vi "Unflatten.vi"(9 "VarTree_in":T1 {"Rawdata" format="0x%08x"}, 11 "In_Char":string) -> (0 "error out":errorcluster, 1 "VarTree_out":T1 {"Rawdata" format="0x%08x"}, 3 "Stat_Ok":bool)   [LabVIEW 2014]
uses:
  _init_vartree/typedefs/ExVarTreeArray.ctl
  _init_vartree/typedefs/ExVarTree.ctl
  _init_vartree/typedefs/val_type_t.ctl
panel:
  out "VarTree size(s)":i32
  out "Read size(s)":i32
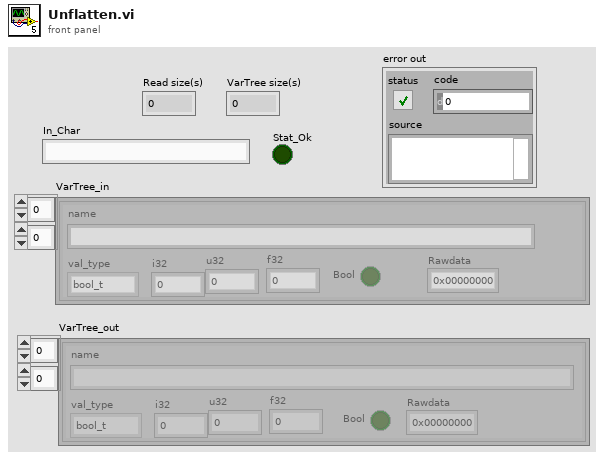
[diagram p1: front panel]
types:
  T1 = typedef "ExVarTreeArray.ctl" = T2[][]
  T2 = typedef "ExVarTree.ctl" = cluster{"name":string, "val_type":T3, "Rawdata":u32, "i32":i32, "u32":u32, "f32":sgl, "Bool":bool}
  T3 = typedef "val_type_t.ctl" = enum16{"bool_t", "i32_t", "u32_t", "f32_t"}
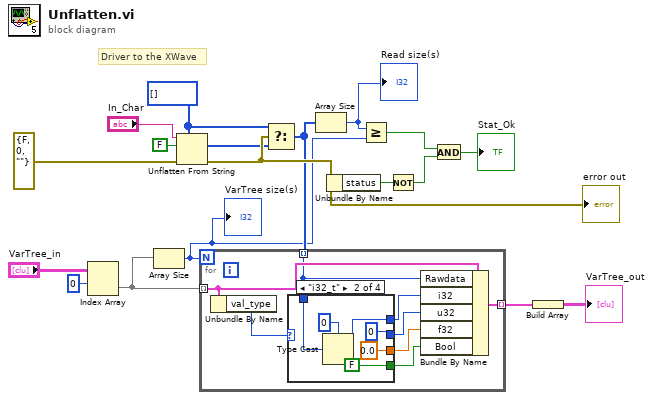
[diagram p0: block diagram]
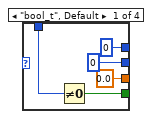
[diagram p2: hidden frame]
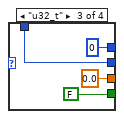
[diagram p3: hidden frame]
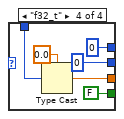
[diagram p4: hidden frame]
diagram:
  w11 = u32[] [] ("sysvars")
  # "Driver to the XWave"
  n1 = Index Array(array="VarTree_in", index (row)=0) -> (element=w12:T2[])  [unwired: 1 in]
  n2 = Array Size(array=w12) -> (size(s)=w5:i32)
  "VarTree size(s)" <- w5
  n3 = Unflatten From String(type=w11, binary string="In_Char", data includes array or string size? (T)=FALSE, error in (no error)=errorcluster {"status"=FALSE, "code"=0, "source"=""}) -> (value=w9:u32[], error out=w18:errorcluster)  [unwired: 1 in, 1 out]
  "error out" <- w18
  n4 = Select(t=w11, s=w18, f=w9) -> (s? t:f=w7:u32[])
  n5 = for {
    N: w5 -> [_]
    tunnel: w7 -> [w23] mode=indexing
    tunnel: w12 -> [w25] mode=indexing
    tunnel: [w26] -> w16 mode=indexing
    n6 = Unbundle By Name(w25) -> ("val_type"=w24:T3)
    n7 = case shown="\"i32_t\"" w24 {
      tunnel: w23 -> [w31 w37 w41 w45]
      tunnel: [0 w35 0 0] -> w22
      tunnel: [u32 0 u32 0 w41 u32 0] -> w21
      tunnel: [sgl 0.0 sgl 0.0 sgl 0.0 w46] -> w20
      tunnel: [w30 FALSE FALSE FALSE] -> w19
      frame "bool_t", Default {
        n8 = Not Equal To 0?(x=w31) -> (x != 0?=w30:bool)
      }
      frame "i32_t" {
        n9 = Type Cast(type=0, x=w37) -> (*(type *) &x=w35:i32)
      }
      frame "u32_t" {
      }
      frame "f32_t" {
        n10 = Type Cast(type=sgl 0.0, x=w45) -> (*(type *) &x=w46:sgl)
      }
    }
    n11 = Bundle By Name(cluster=w25, "Rawdata"=w23, "i32"=w22, "u32"=w21, "f32"=w20, "Bool"=w19) -> (w26:T2)
  }
  n12 = Array Size(array=w7) -> (size(s)=w6:i32)
  "Read size(s)" <- w6
  n13 = Unbundle By Name(w18) -> ("status"=w1:bool)
  n14 = Greater Or Equal?(x=w6, y=w5) -> (x >= y?=w4:bool)
  n15 = Not(x=w1) -> (.not. x?=w2:bool)
  n16 = And(x=w4, y=w2) -> (x .and. y?=→"Stat_Ok":bool)
  n17 = Build Array(w16) -> (→"VarTree_out":T2[][])
